vi "Init Events.vi"(8 "error in (no error)":errorcluster, 11 "AppListPanel in":refnum<class "AppListPanel.lvclass">) -> (0 "error out":errorcluster, 3 "AppListPanel out":refnum<class "AppListPanel.lvclass">)   [LabVIEW 2020, in "PicoG-App.lvlib" / "AppListPanel.lvclass"]
uses:
  AppListPanel.lvclass
  ViaApp/ViaApp.lvclass
  AppListPanel.lvclass/AppListPanel.ctl
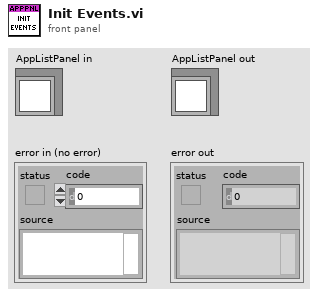
[diagram p1: front panel]
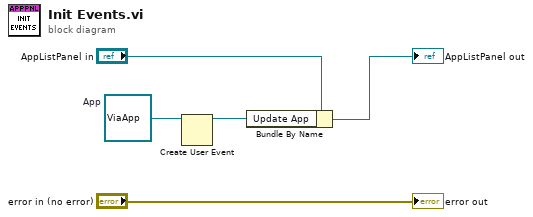
[diagram p0: block diagram]
diagram:
  w2 = refnum<class "ViaApp.lvclass"> refnum  # App
  n1 = Create User Event(user event datatype=w2) -> (user event=w1:refnum<user-event>)  [unwired: 1 in, 1 out]
  n2 = Bundle By Name(cluster="AppListPanel in", "Update App"=w1) -> (→"AppListPanel out":refnum<class "AppListPanel.lvclass">)
  "error out" <- "error in (no error)"
